vi "Configure Sweep Mode.vi"(8 "error in (no error)":errorcluster, 10 "Sweep Mode":enum16{"Continuous", "Single"}(ring), 11 "MXA in":refnum<class "MXA.lvclass">) -> (0 "error out":errorcluster, 3 "MXA out":refnum<class "MXA.lvclass">)   [LabVIEW 2020, in "MXA.lvclass"]
uses:
  MXA.lvclass
  C:/Sandbox/RF Bench/Source Code/WiSpry Test Framework/Instruments/Instrument.lvclass
  Instrument.lvclass/Instrument.ctl
  Instrument.lvclass
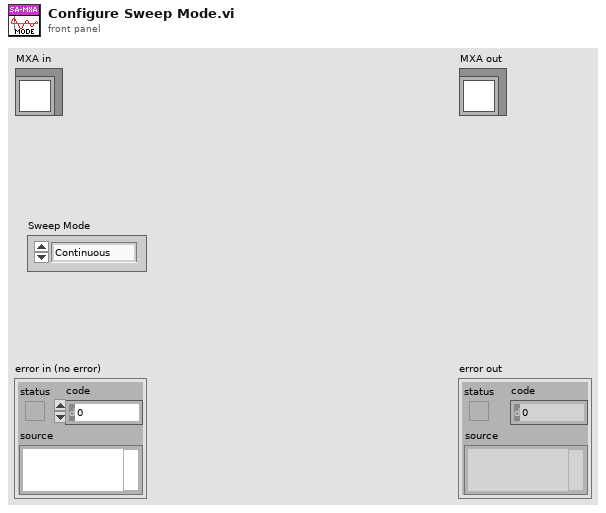
[diagram p1: front panel]
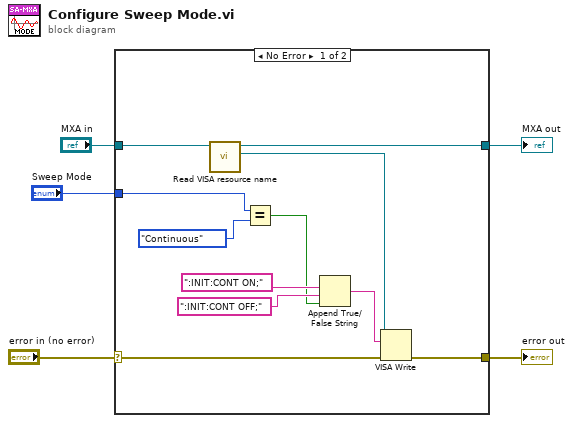
[diagram p0: block diagram]
diagram:
  n1 = case shown="No Error" "error in (no error)" {
    selector: "error in (no error)" -> [w7 w18]
    tunnel: "MXA in" -> [w16 w17]
    tunnel: [w8 w18] -> w5
    tunnel: [w15 w17] -> w4
    tunnel: "Sweep Mode" -> [w10 _]
    frame No Error {
      n2 = call "Read VISA resource name.vi"("Instrument in"=w16) -> ("VISA resource name"=w6:refnum<visa-resource-name>, "Instrument out"=w15:refnum<class "MXA.lvclass">)  [unwired: 9 in]
      n3 = Equal?(x=w10, y=enum16{"Continuous", "Single"}."Continuous" ("Sweep Mode")) -> (x = y?=w9:bool)
      n4 = Append True/False String(1:w9, 2:":INIT:CONT OFF;" ("false string"), 3:":INIT:CONT ON;" ("format string")) -> (0:w12:string)  [unwired: 1 in]
      n5 = VISA Write(VISA resource name=w6, write buffer=w12, error in (no error)=w7) -> (error out=w8:errorcluster)  [unwired: 2 out]
    }
    frame Error {
    }
  }
  "error out" <- w5
  "MXA out" <- w4
